vi "On Save As UI Showing.vi"(8 "error in (no error)":errorcluster, 10 "ContentMimeType":string, 11 "WebView2 Event Filter Interface in":refnum<class "WebView2 Event Filter Interface.lvclass">) -> (0 "error out":errorcluster, 2 "Response":T1 {"Kind" items=["Default", "HtmlOnly", "SingleFile", "Complete"]})   [LabVIEW 2025, in "WebView2.lvlib" / "WebView2 Event Filter Interface.lvclass"]
uses:
  WebView2 Event Filter Interface.lvclass
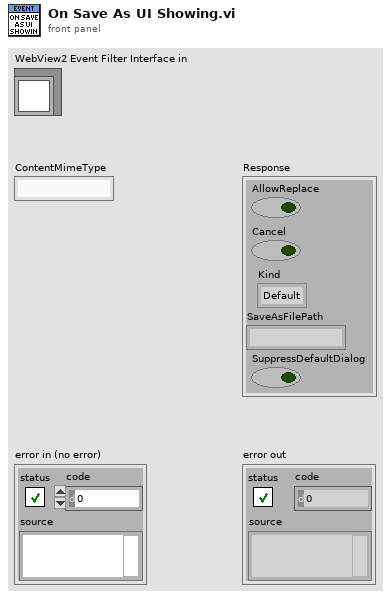
[diagram p1: front panel]
types:
  T1 = cluster{"AllowReplace":bool, "Cancel":bool, "Kind":i32, "SaveAsFilePath":string, "SuppressDefaultDialog":bool}
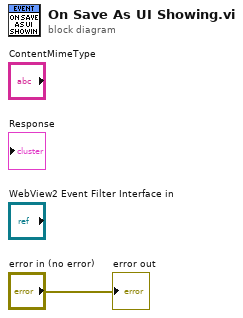
[diagram p0: block diagram]
diagram:
  "error out" <- "error in (no error)"
